vi "subtract.vi"(1 "b":dbl, 2 "a":dbl) -> (0 "result":dbl)   [LabVIEW 2019, in "lv-providershell-example1.lvlib"]
uses:
  lv-providershell-example1.lvlib
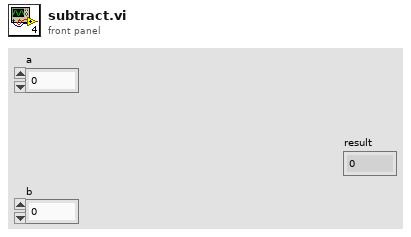
[diagram p1: front panel]
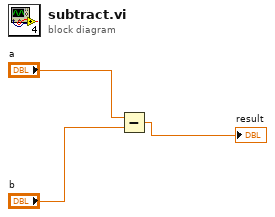
[diagram p0: block diagram]
diagram:
  n1 = Subtract(x="a", y="b") -> (x-y=→"result":dbl)
